vi "Scannvorgang_Ellipse.vi"(2 "Sweep":dbl[](array[numeric])=array[10000 elements], 3 "Sequenz length us":i32=10000, 8 "aktuelle z_wagen":dbl=37.06357865384881, 9 "aktuelle x_wagen":dbl=94.93642134615119, 10 "z_Ellipse":i32=40, 11 "x_Ellipse":u8=110 max=200 step=1) -> (1 "Maximale Gap":dbl=73.92227807370318)   [LabVIEW 2014]
panel:
  out "Schrittweite (° )":dbl=17.33884931601344 format="%#_13g"
  in  "Registerkarte":enum32{"Seite 1", "Seite 2"}(tab)
  in  "Schrittweite (°)\nbeim scannen":dbl=1.8 min=0.8999999761581421 max=180.0 step=0.1
  out "Welche Mikrofon arbeitet":tag="Dev2/ai2"
  out "IR with theshold":dbl[][](graph)
  out "Peak Locations":dbl[](array[numeric])=[1411.7792219498556, 1485.4707888222586, 1553.4812108242002]
  out "Gap":dbl=73.69156687240297
  out "Wahrscheinlichkeit":dbl=0.18180011321187692
  out "Gaparray":dbl[](array[numeric])=[0.0, 0.0, 0.0, 70.40982015794248, 73.9825353555093, 93.77119367083696, 89.1289817011259, 86.33413922941645, 71.46893395154802, 71.70369857274227, 71.69078916281705, 71.78635788746942, 72.704362947743, 71.7352662484152, 73.92227807370318, 79.18330937111, 74.47469247457639, 73.69156687240297]
  out "Wahrscheinlichkeit*Apulitude":dbl[](array[numeric])=[0.0, 0.0, 0.0, 0.34958454259626265, 59.83804534701513, 5.2884704340977004e-33, 3.3145426239114387e-18, 3.8952884609568596e-11, 17.93564797575579, 51.21969373366334, 104.30933663252114, 141.63230883320028, 465.1572957491611, 131.2560263527799, 774.8792832882529, 6.127297906295946, 253.85308786269772, 89.48591059763186]
  out "Welche LS arbeitet":i32=4
  out "Maximale Gap gefunde?":bool
  out "Anzahl des Scannvorgang":i32=2
  out "Max. Index":i32=14
  out "Winkel_zurück drehen":dbl=27.0
  out "Schrittweite rechnen (° )":dbl=27.0 format="%#_13g"
  out "Abstatnd in mm":dbl=238.45926955595573
  out "z_Ellipse>100?":bool
  in  "RN-Motor - RS232":refnum<visa-resource-name>="COM5"
  in  "Motor an?":bool=TRUE
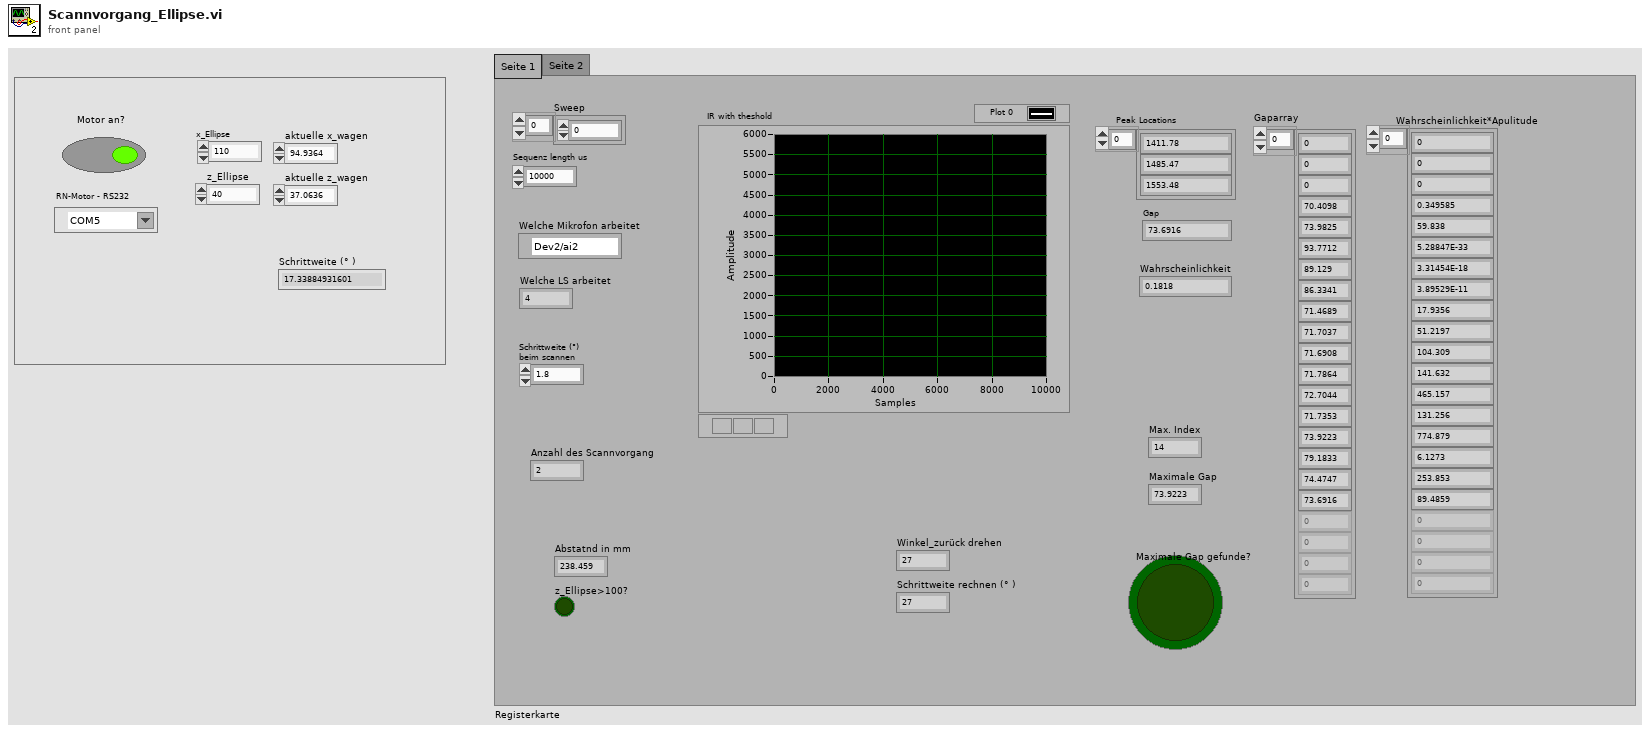
[diagram p1: front panel]
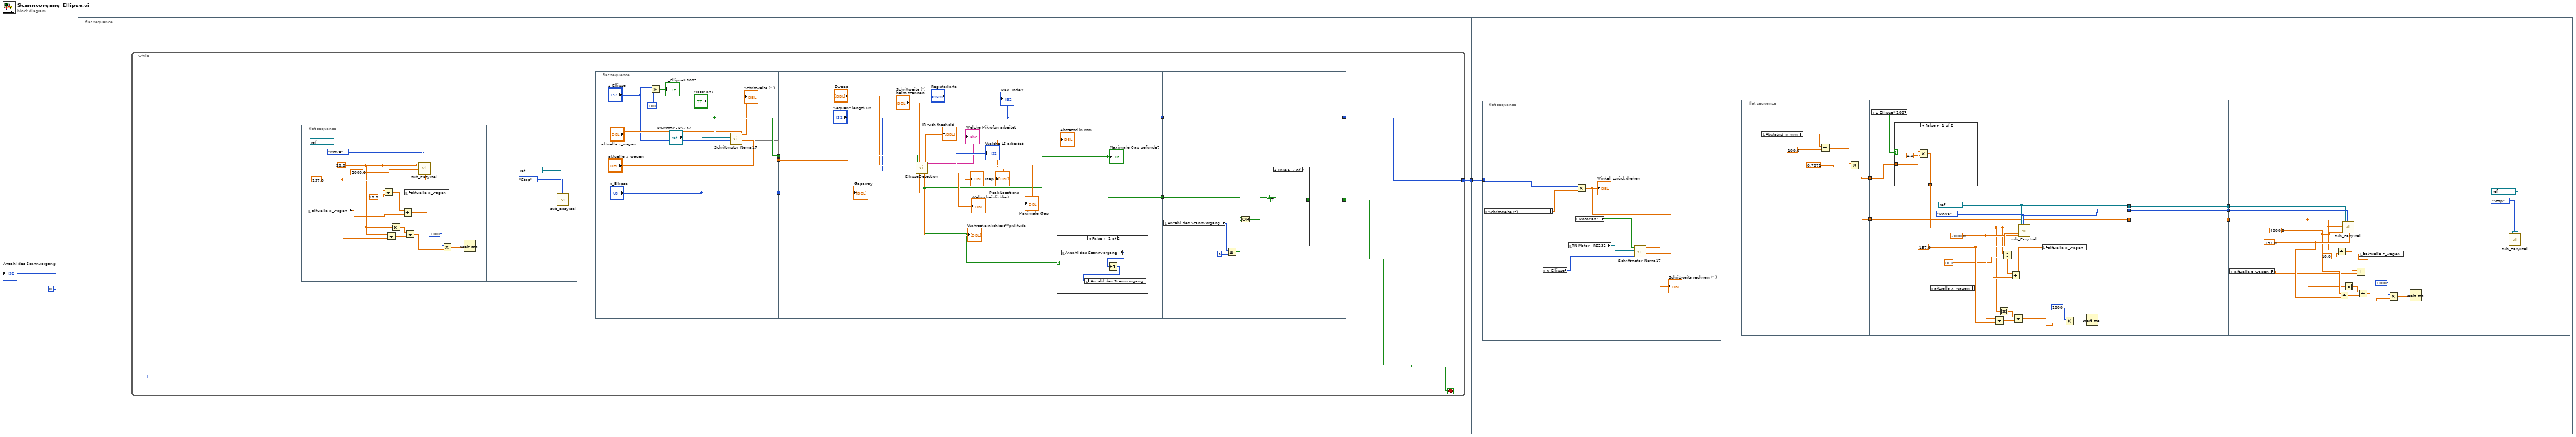
[diagram p0: block diagram]
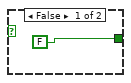
[diagram p3: hidden frame]
diagram:
  n1 = flat-sequence {
    tunnel: [w3] -> w1
    tunnel: w1 -> [w66]
    frame #0 {
      n2 = while {
        tunnel: [w8] -> w3
        stop <- w4 stop-if-true
        n3 = flat-sequence {
          frame #0 {
            w11 = 20.0 ("x-Position")
            w15 = 157.0 ("Steps/mm (z)")
            n4 = local read "aktuelle x_wagen"() -> (w21:dbl)
            n5 = Divide(x=w11, y=10.0 ("x/y")) -> (x/y=w18:dbl)
            n6 = Divide(x=w11, y=w15) -> (x/y=w16:dbl)
            n7 = Absolute Value(x=w11) -> (abs(x)=w17:dbl)
            n8 = Add(x=w18, y=w21) -> (x+y=w22:dbl)
            n9 = Divide(x=w17, y=w16) -> (x/y=w14:dbl)
            n10 = local write "aktuelle x_wagen"(w22) -> ()
            n11 = call "sub_EasyIsel.vi"("x-Position"=w11, "Velocity (x)"=2000.0, "VISA resource name"=refnum<visa-resource-name> "COM4", "Mode"=enum16{"Position", "Move", "Stop", "Home"}."Move", "Steps/mm (z)"=w15) -> ()  [unwired: 11 in, 4 out]
            n12 = Multiply(x=u32 1000 ("Zu wartende ms"), y=w14) -> (x*y=w24:dbl)
            n13 = Wait (ms)(milliseconds to wait=w24) -> ()  [unwired: 1 out]
          }
          frame #1 {
            n14 = call "sub_EasyIsel.vi"("VISA resource name"=refnum<visa-resource-name> "COM4", "Mode"=enum16{"Position", "Move", "Stop", "Home"}."Stop") -> ()  [unwired: 14 in, 4 out]
          }
        }
        n15 = flat-sequence {
          tunnel: ["Motor an?"] -> w10
          tunnel: ["x_Ellipse"] -> w9
          tunnel: [w31] -> w7
          tunnel: w10 -> [w45]
          tunnel: w9 -> [w42]
          tunnel: w7 -> [w39]
          tunnel: [w41] -> w6
          tunnel: [w38] -> w5
          tunnel: [w63] -> w8
          tunnel: w6 -> [w63]
          tunnel: w5 -> [w58]
          tunnel: [w62] -> w4
          frame #0 {
            n16 = Greater Or Equal?(x="z_Ellipse", y=100) -> (x >= y?=→"z_Ellipse>100?":bool)
            n17 = call "Schrittmotor_Nema17.vi"(0:"aktuelle z_wagen", "Schrittweite  eingeben"="aktuelle x_wagen", "x_Ellipse"="x_Ellipse", 9:"z_Ellipse", "RN-Motor - RS232 2"="RN-Motor - RS232", "Motor an?"="Motor an?") -> ("Schrittweite rechnen"=→"Schrittweite (° )":dbl, 6:w31)  [unwired: 4 in]
          }
          frame #1 {
            n18 = call "EllipseDetection.vi"("Motor an?"=w45, "Sweep"="Sweep", "Winkel_ende"=w39, "Sequenz length us"="Sequenz length us", "x_Ellipse"=w42, "Schrittweite (°)"="Schrittweite (°)\nbeim scannen") -> ("Gaparray"=→"Gaparray":dbl[], "Max. Index"=w41:i32, "Maximale Gap"=→"Maximale Gap":dbl, "Wahrscheinlichkeit*Apulitude"=→"Wahrscheinlichkeit*Apulitude":dbl[], "IR with theshold"=→"IR with theshold":dbl[][], "Maximale Gap gefunde?"=w38:bool, "Welche Mikrofon arbeitet"=→"Welche Mikrofon arbeitet":tag, "Welche LS arbeitet"=→"Welche LS arbeitet":i32, "Abstatnd"=→"Abstatnd in mm":dbl, "Peak Locations"=→"Peak Locations":dbl[], "Gap"=→"Gap":dbl, "Wahrscheinlichkeit"=→"Wahrscheinlichkeit":dbl)  [unwired: 2 in]
            "Maximale Gap gefunde?" <- w38
            "Max. Index" <- w41
            n19 = case shown="False" w38 {
              frame False {
                n20 = local read "Anzahl des Scannvorgang"() -> (w56:i32)
                n21 = Increment(x=w56) -> (x+1=w55:i32)
                n22 = local write "Anzahl des Scannvorgang"(w55) -> ()
              }
              frame True {
              }
            }
          }
          frame #2 {
            n23 = local read "Anzahl des Scannvorgang"() -> (w60:i32)
            n24 = Greater Or Equal?(x=w60, y=3) -> (x >= y?=w59:bool)
            n25 = Or(x=w58, y=w59) -> (x .or. y?=w57:bool)
            n26 = case shown="True" w57 {
              tunnel: [FALSE TRUE] -> w62
              frame False {
              }
              frame True {
              }
            }
          }
        }
      }
    }
    frame #1 {
      n27 = flat-sequence {
        tunnel: w66 -> [w67]
        frame #0 {
          n28 = local read "Schrittweite (°)\nbeim scannen"() -> (w73:dbl)
          n29 = local read "x_Ellipse"() -> (w69:u8)
          n30 = local read "RN-Motor - RS232"() -> (w71:refnum<visa-resource-name>)
          n31 = local read "Motor an?"() -> (w72:bool)
          n32 = Multiply(x=w67, y=w73) -> (x*y=w70:dbl)
          "Winkel_zurück drehen" <- w70
          n33 = call "Schrittmotor_Nema17.vi"("Schrittweite  eingeben"=w70, "x_Ellipse"=w69, "RN-Motor - RS232 2"=w71, "Motor an?"=w72) -> ("Schrittweite rechnen"=→"Schrittweite rechnen (° )":dbl)  [unwired: 7 in]
        }
      }
    }
    frame #2 {
      n34 = flat-sequence {
        tunnel: [w82] -> w81
        tunnel: [w82] -> w80
        tunnel: w81 -> [w90]
        tunnel: [w92] -> w79
        tunnel: [w91] -> w77
        tunnel: [w90] -> w75
        tunnel: w80 -> [w88]
        tunnel: w79 -> [w110]
        tunnel: [w110] -> w78
        tunnel: w77 -> [w109]
        tunnel: [w109] -> w76
        tunnel: w75 -> [w108]
        tunnel: [w108] -> w74
        tunnel: w78 -> [w115]
        tunnel: w76 -> [w114]
        tunnel: w74 -> [w111]
        frame #0 {
          n35 = local read "Abstatnd in mm"() -> (w86:dbl)
          n36 = Subtract(x=w86, y=100.0) -> (x-y=w84:dbl)
          n37 = Multiply(x=w84, y=0.7071) -> (x*y=w82:dbl)
        }
        frame #1 {
          w91 = refnum<visa-resource-name> "COM4" ("VISA resource name")
          w92 = enum16{"Position", "Move", "Stop", "Home"}."Move" ("Mode")
          w103 = 157.0 ("Steps/mm (z)")
          w102 = 2000.0 ("Velocity (z)")
          n38 = local read "z_Ellipse>100?"() -> (w89:bool)
          n39 = case shown="False" w89 {
            tunnel: w88 -> [w106 w107]
            tunnel: [w104 w107] -> w87
            frame False {
              n40 = Multiply(x=w106, y=-1.0) -> (x*y=w104:dbl)
            }
            frame True {
            }
          }
          n41 = local read "aktuelle x_wagen"() -> (w95:dbl)
          n42 = Divide(x=w102, y=w103) -> (x/y=w101:dbl)
          n43 = Absolute Value(x=w87) -> (abs(x)=w100:dbl)
          n44 = Divide(x=w87, y=10.0 ("x/y")) -> (x/y=w99:dbl)
          n45 = Add(x=w99, y=w95) -> (x+y=w94:dbl)
          n46 = Divide(x=w100, y=w101) -> (x/y=w93:dbl)
          n47 = call "sub_EasyIsel.vi"("x-Position"=w87, "Velocity (z)"=w102, "VISA resource name"=w91, "Mode"=w92, "Steps/mm (z)"=w103) -> ()  [unwired: 11 in, 4 out]
          n48 = local write "aktuelle x_wagen"(w94) -> ()
          n49 = Multiply(x=u32 1000 ("Zu wartende ms"), y=w93) -> (x*y=w96:dbl)
          n50 = Wait (ms)(milliseconds to wait=w96) -> ()  [unwired: 1 out]
        }
        frame #2 {
        }
        frame #3 {
          w124 = 157.0 ("Steps/mm (z)")
          w123 = 4000.0 ("Velocity (z)")
          n51 = local read "aktuelle z_wagen"() -> (w112:dbl)
          n52 = Divide(x=w111, y=10.0 ("x/y")) -> (x/y=w120:dbl)
          n53 = Divide(x=w123, y=w124) -> (x/y=w122:dbl)
          n54 = call "sub_EasyIsel.vi"("z-Position"=w111, "Velocity (z)"=w123, "VISA resource name"=w114, "Mode"=w115, "Steps/mm (z)"=w124) -> ()  [unwired: 11 in, 4 out]
          n55 = Absolute Value(x=w111) -> (abs(x)=w121:dbl)
          n56 = Add(x=w120, y=w112) -> (x+y=w113:dbl)
          n57 = Divide(x=w121, y=w122) -> (x/y=w116:dbl)
          n58 = local write "aktuelle z_wagen"(w113) -> ()
          n59 = Multiply(x=u32 1000 ("Zu wartende ms"), y=w116) -> (x*y=w117:dbl)
          n60 = Wait (ms)(milliseconds to wait=w117) -> ()  [unwired: 1 out]
        }
        frame #4 {
          n61 = call "sub_EasyIsel.vi"("VISA resource name"=refnum<visa-resource-name> "COM4", "Mode"=enum16{"Position", "Move", "Stop", "Home"}."Stop") -> ()  [unwired: 14 in, 4 out]
        }
      }
    }
  }
  "Anzahl des Scannvorgang" <- 0 ("Anzahl des Scannvorgang")
